vi "EEI EXP4.vi"() -> ()   [LabVIEW 2020]
panel:
  in  "Numeric3":i32
  out "Numeric":i32
  out "current time":timestamp
  out "Sum using for loop":i32
  in  "N value":i32
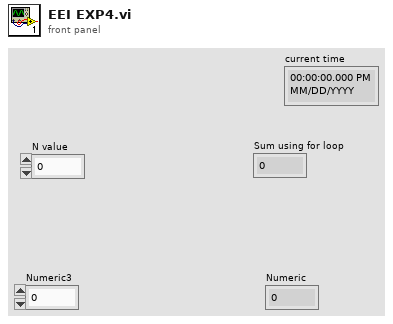
[diagram p1: front panel]
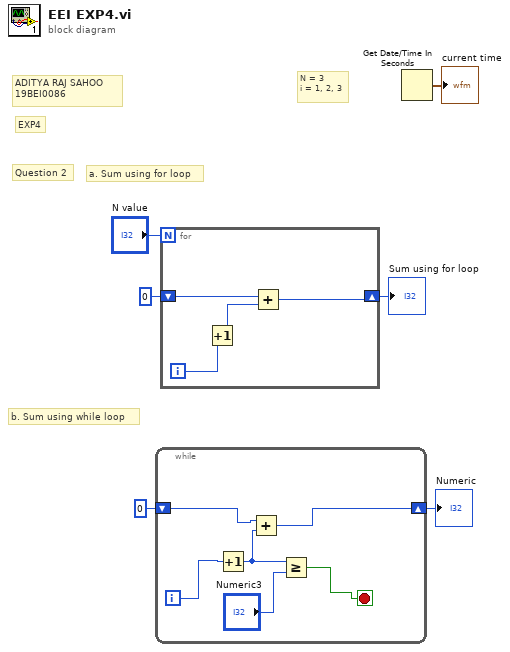
[diagram p0: block diagram]
diagram:
  # "EXP4"
  # "b. Sum using while loop"
  # "a. Sum using for loop"
  # "ADITYA RAJ SAHOO\n19BEI0086"
  # "Question 2"
  # "N = 3\ni = 1, 2, 3"
  n1 = while {
    shift-right: [w11] -> w1
    shift-left: 0 -> [w12]
    i -> [w10]
    stop <- w9 stop-if-true
    n2 = Increment(x=w10) -> (x+1=w8:i32)
    n3 = Add(x=w12, y=w8) -> (x+y=w11:i32)
    n4 = Greater Or Equal?(x=w8, y="Numeric3") -> (x >= y?=w9:bool)
  }
  "Numeric" <- w1
  n5 = for {
    N: "N value" -> [_]
    shift-right: [w13] -> w4
    shift-left: 0 -> [w14]
    i -> [w16]
    n6 = Increment(x=w16) -> (x+1=w15:i32)
    n7 = Add(x=w14, y=w15) -> (x+y=w13:i32)
  }
  "Sum using for loop" <- w4
  n8 = Get Date/Time In Seconds() -> (seconds since 1Jan1904=→"current time":timestamp)
